vi "Get Name.vi"(8 "error in (no error)":errorcluster, 11 "DD Parent in":refnum<class "DD Parent.lvclass">) -> (0 "error out":errorcluster, 2 "name":string, 3 "DD Parent out":refnum<class "DD Parent.lvclass">)   [LabVIEW 2016, in "DD Parent.lvclass"]
uses:
  DD Parent.lvclass
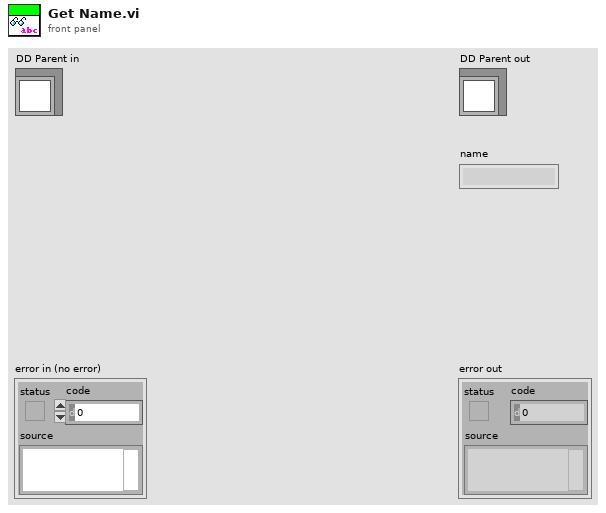
[diagram p1: front panel]
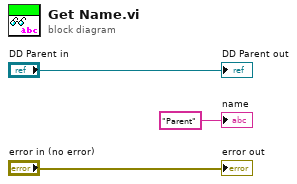
[diagram p0: block diagram]
diagram:
  "error out" <- "error in (no error)"
  "DD Parent out" <- "DD Parent in"
  "name" <- "Parent" ("name")
